vi "WORD report.vi"(7 "Action":T1=enum."Close report", 8 "error in":errorcluster, 10 "Data in":string) -> (0 "error out":errorcluster, 2 "Data out":variant)   [LabVIEW 2016, in "Report.lvlib"]
uses:
  Report.lvlib
  TypeDefs/Report state.ctl
  TypeDefs/Report data.ctl
  <vilib>/Utility/NIReport.llb/NI_report.lvclass
  <vilib>/Utility/NIReport.llb/Append Report Text (str wrap).vi
  <vilib>/Utility/NIReport.llb/NI_ReportGenerationCore.lvlib
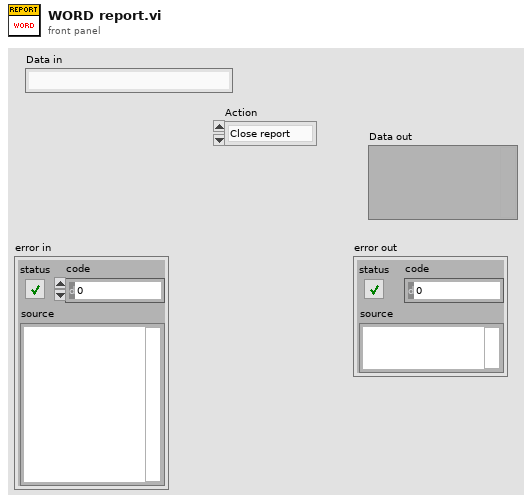
[diagram p1: front panel]
types:
  T1 = typedef "Report.lvlib/Report state.ctl" = enum16{"Create report", "Save data", "Save report", "Available printers", "Print report", "Close report"}
  T2 = enum16{"maximized", "minimized", "normal", "no change"}
  T3 = enum16{"Standard Report", "HTML", "Word", "Excel"}
  T4 = typedef "Report.lvlib/Report data.ctl" = cluster{"report ID":refnum<class "NI_report.lvclass">, "error":errorcluster}
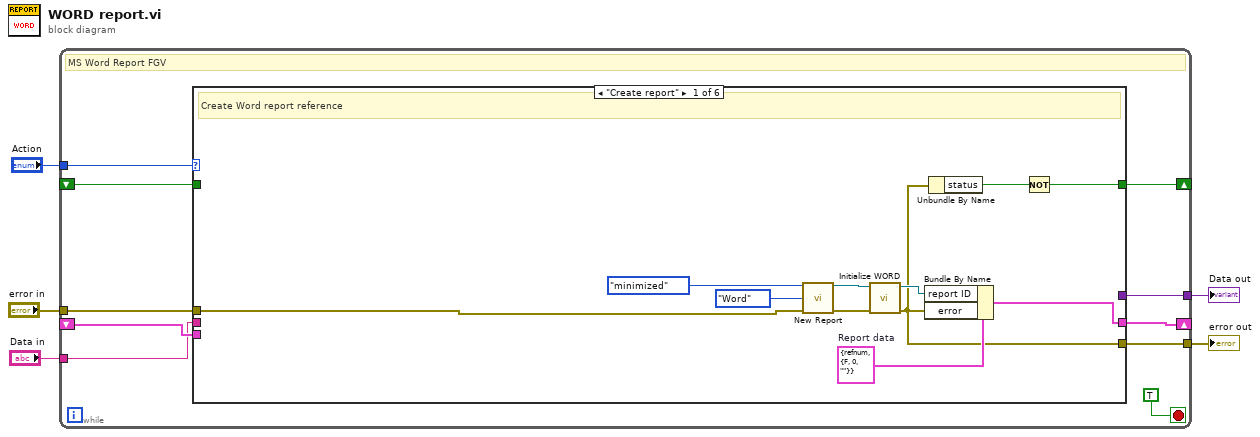
[diagram p0: block diagram]
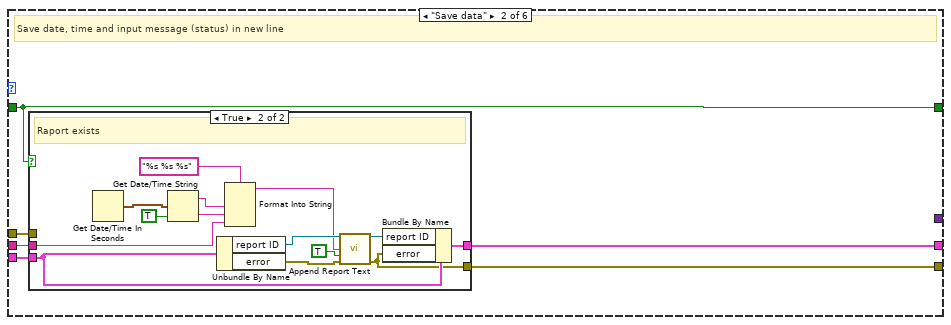
[diagram p2: hidden frame]
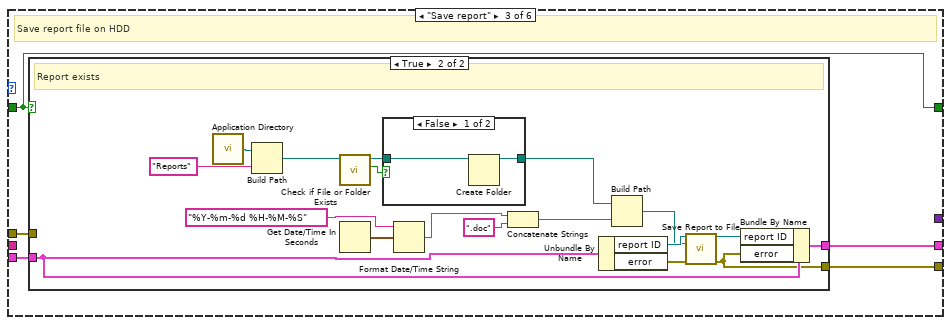
[diagram p4: hidden frame]
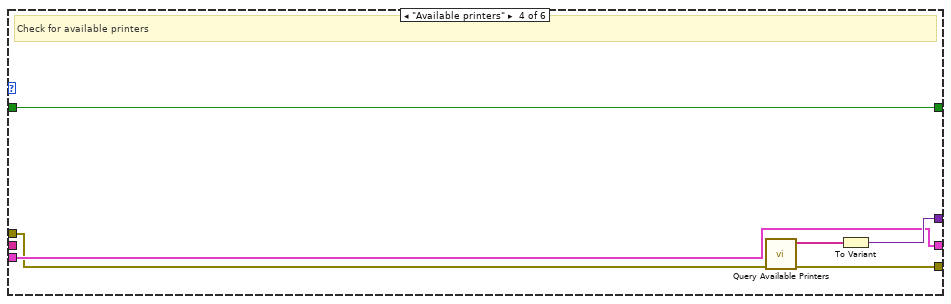
[diagram p7: hidden frame]
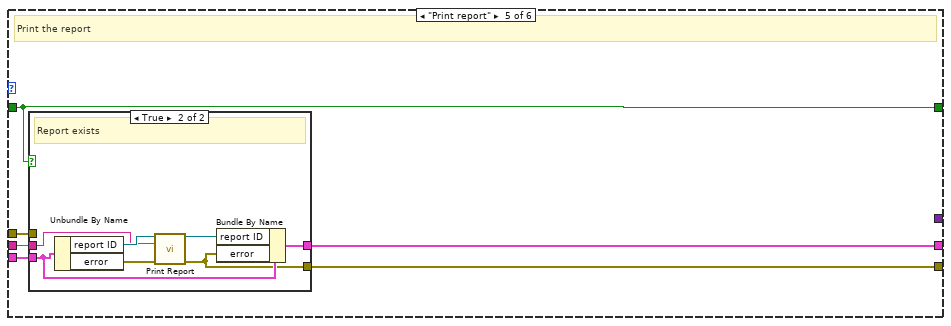
[diagram p8: hidden frame]
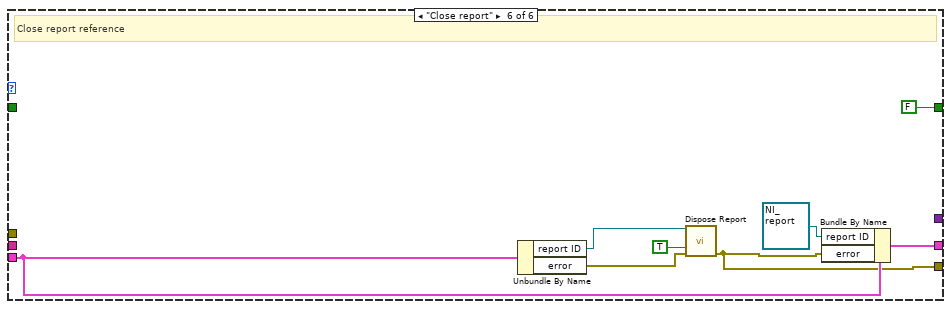
[diagram p10: hidden frame]
diagram:
  n1 = while {
    tunnel: "Action" -> [w11]
    shift-right: [w13] -> _
    shift-left: _ -> [w14]
    tunnel: "Data in" -> [w12]
    tunnel: "error in" -> [w10]
    tunnel: [w9] -> w3
    tunnel: [w8] -> w1
    shift-right: [w6] -> _
    shift-left: _ -> [w7]
    stop <- TRUE stop-if-true
    # "MS Word Report FGV"
    n2 = case shown="\"Create report\"" w11 {
      tunnel: w14 -> [_ w32 w53 w80 w88 w104]
      tunnel: [w26 w31 w52 w80 w87 w105] -> w13
      tunnel: w12 -> [_ w30 _ _ w86 _]
      tunnel: w10 -> [w19 w27 w49 w79 w83 _]
      tunnel: [_ _ _ w81 _ _] -> w9
      tunnel: [w18 w29 w51 w78 w85 w100] -> w8
      tunnel: w7 -> [_ w28 w50 w77 w84 _]
      tunnel: [w16 w28 w50 w77 w84 FALSE] -> w6
      frame "Create report" {
        w20 = T4 {"report ID"=refnum, "error"={"status"=FALSE, "code"=0, "source"=""}}  # Report data
        # "Create Word report reference"
        n3 = call <vilib>:"New Report.vi"("window state (normal)"=T2."minimized", "report type"=T3."Word", "error in (no error)"=w19) -> ("report out"=w23:refnum<class "NI_report.lvclass">, "error out"=w22:errorcluster)  [unwired: 11 in]
        n4 = call "Initialize WORD.vi"("error in (no error)"=w22, "NI_report in"=w23) -> ("error out"=w18:errorcluster, "NI_report out"=w21:refnum<class "NI_report.lvclass">)  [unwired: 8 in]
        n5 = Bundle By Name(cluster=w20, "report ID"=w21, "error"=w18) -> (w26:T4)
        n6 = Unbundle By Name(w18) -> ("status"=w17:bool)
        n7 = Not(x=w17) -> (.not. x?=w16:bool)
      }
      frame "Save data" {
        # "Save date, time and input message (status) in new line"
        n8 = case shown="True" w28 {
          tunnel: w32 -> [w33 w46]
          tunnel: [w33 w44] -> w31
          tunnel: w30 -> [_ w36]
          tunnel: [w34 w35] -> w29
          tunnel: w27 -> [w34 _]
          frame False {
            # "Report not created"
          }
          frame True {
            # "Raport exists"
            n9 = Get Date/Time In Seconds() -> (seconds since 1Jan1904=w42:timestamp)
            n10 = Get Date/Time String(seconds (now)=w42, want seconds? (F)=TRUE) -> (date string=w40:string, time string=w39:string)  [unwired: 1 in]
            n11 = Unbundle By Name(w46) -> ("report ID"=w48:refnum<class "NI_report.lvclass">, "error"=w47:errorcluster)
            n12 = Format Into String(format string="%s %s %s", w40, w39, w36) -> (resulting string=w37:string)  [unwired: 2 in, 1 out]
            n13 = call-poly <vilib>:"Append Report Text.vi"("report in"=w48, "text"=w37, "append on new line? (F)"=TRUE, "error in (no error)"=w47) -> ("report out"=w45:refnum<class "NI_report.lvclass">, "error out"=w35:errorcluster)  [unwired: 8 in, 2 out]
            n14 = Bundle By Name(cluster=w46, "report ID"=w45, "error"=w35) -> (w44:T4)
          }
        }
      }
      frame "Save report" {
        # "Save report file on HDD"
        n15 = case shown="True" w50 {
          tunnel: w53 -> [w55 w73]
          tunnel: [w55 w72] -> w52
          tunnel: [w54 w56] -> w51
          tunnel: w49 -> [w54 _]
          frame False {
            # "Report not created"
          }
          frame True {
            # "Report exists"
            n16 = call <vilib>:"Application Directory.vi"() -> ("Application Directory"=w62:path)
            n17 = Build Path(base path=w62, name or relative path="Reports") -> (appended path=w60:path)
            n18 = call <vilib>:"Check if File or Folder Exists.vi"("path"=w60) -> ("file or folder exists?"=w59:bool, "dup path"=w58:path)  [unwired: 8 in, 1 out]
            n19 = Get Date/Time In Seconds() -> (seconds since 1Jan1904=w67:timestamp)
            n20 = case shown="False" w59 {
              tunnel: w58 -> [w75 w76]
              tunnel: [w74 w76] -> w57
              frame False {
                n21 = Create Folder(path (use dialog)=w75) -> (created path=w74:path)  [unwired: 2 in, 2 out]
              }
              frame True {
              }
            }
            n22 = Format Date/Time String(time format string (%c)="%Y-%m-%d %H-%M-%S", seconds (now)=w67) -> (date/time string=w65:string)  [unwired: 1 in]
            n23 = Concatenate Strings(w65, ".doc" ("string")) -> (w63:string)
            n24 = Unbundle By Name(w73) -> ("report ID"=w71:refnum<class "NI_report.lvclass">, "error"=w70:errorcluster)
            n25 = Build Path(base path=w57, name or relative path=w63) -> (appended path=w68:path)
            n26 = call-dynamic "Save Report to File.vi"("report in"=w71, "report file path"=w68, "error in (no error)"=w70) -> ("report out"=w69:refnum<class "NI_report.lvclass">, "error out"=w56:errorcluster)  [unwired: 11 in]
            n27 = Bundle By Name(cluster=w73, "report ID"=w69, "error"=w56) -> (w72:T4)
          }
        }
      }
      frame "Available printers" {
        # "Check for available printers"
        n28 = call <vilib>:"Query Available Printers.vi"("error in (no error)"=w79) -> ("error out"=w78:errorcluster, "system configured printers"=w82:string[])  [unwired: 8 in, 1 out]
        n29 = To Variant(anything=w82) -> (Variant=w81:variant)
      }
      frame "Print report" {
        # "Print the report"
        n30 = case shown="True" w84 {
          tunnel: w88 -> [w89 w95]
          tunnel: [w89 w94] -> w87
          tunnel: w86 -> [_ w92]
          tunnel: [w90 w91] -> w85
          tunnel: w83 -> [w90 _]
          frame False {
            # "Report not created"
          }
          frame True {
            # "Report exists"
            n31 = Unbundle By Name(w95) -> ("report ID"=w97:refnum<class "NI_report.lvclass">, "error"=w96:errorcluster)
            n32 = call-dynamic "Print Report.vi"("report in"=w97, "printer name (default)"=w92, "error in (no error)"=w96) -> ("report out"=w93:refnum<class "NI_report.lvclass">, "error out"=w91:errorcluster)  [unwired: 11 in]
            n33 = Bundle By Name(cluster=w95, "report ID"=w93, "error"=w91) -> (w94:T4)
          }
        }
      }
      frame "Close report" {
        # "Close report reference"
        n34 = Unbundle By Name(w104) -> ("report ID"=w103:refnum<class "NI_report.lvclass">, "error"=w102:errorcluster)
        n35 = call-dynamic "Dispose Report.vi"("report in"=w103, "save changes? (F)"=TRUE, "error in (no error)"=w102) -> ("error out"=w100:errorcluster)  [unwired: 12 in]
        n36 = Bundle By Name(cluster=w104, "report ID"=refnum<class "NI_report.lvclass"> refnum, "error"=w100) -> (w105:T4)
      }
    }
  }
  "error out" <- w1
  "Data out" <- w3
